vi "getPDF.vi"(6 "addr/port":cluster{"address":string, "port":i32}={"address"="127.0.0.1", "port"=31415}, 8 "error in (no error)":errorcluster) -> (0 "error out":errorcluster, 3 "PDF":dbl[](array[numeric]))   [LabVIEW 2015]
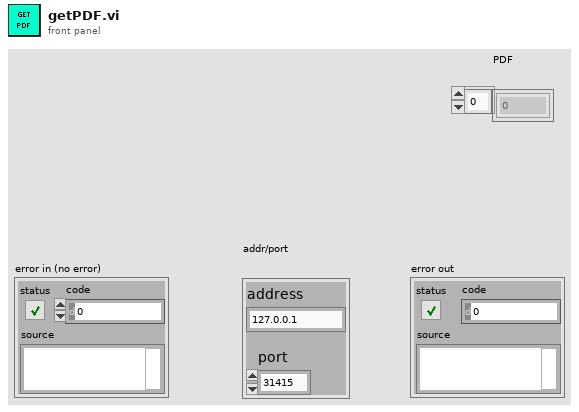
[diagram p1: front panel]
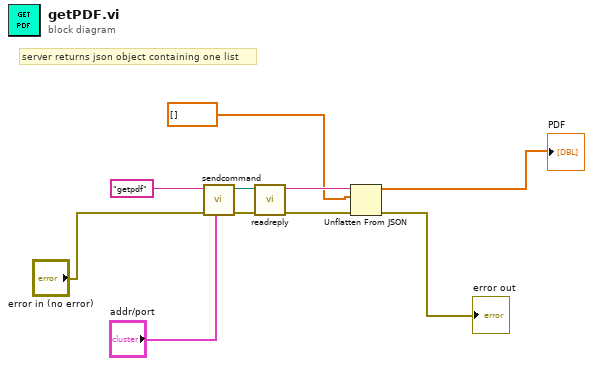
[diagram p0: block diagram]
diagram:
  # "server returns json object containing one list"
  n1 = call "sendcommand.vi"("addr/port"="addr/port", "error in (no error)"="error in (no error)", "command"="getpdf") -> ("error out"=w6:errorcluster, "connection ID out"=w7:refnum<k5>)  [unwired: 6 in, 1 out]
  n2 = call "readreply.vi"("error in (no error)"=w6, "connection ID"=w7) -> ("error out"=w5:errorcluster, "data out"=w3:string)  [unwired: 8 in]
  n3 = Unflatten From JSON(JSON string=w3, type and defaults=dbl[] [] ("Array"), error in (no error)=w5) -> (value=→"PDF":dbl[], error out=→"error out":errorcluster)  [unwired: 4 in]
